vi "Configure Current Limits.vi"(0 "VISA resource name":refnum<visa-resource-name>, 5 "Current Low Limit (0 A)":dbl min=0.0 max=220.8 format="%.3f", 7 "Current High Limit (0 A)":dbl min=0.0 max=220.8 format="%.3f", 9 "Current Type":u16(ring) items=["RMS", "Peak"], 11 "error in (no error)":errorcluster) -> (4 "VISA resource name out":refnum<visa-resource-name>, 15 "error out":errorcluster)   [LabVIEW 2016, in "APT 300XAC Series.lvlib"]
doc: "Configure the current limits in the active step of the power source instrument.\n\n<B>Range</B> : 0.000~55.20 A\n\nAC Mode\nVoltage Range = Low\n310XAC=0.000-9.20\n320XAC=0.000-18.40\n340XAC=0.00-36.80\n360XAC=0.00-55.20\n\nVoltage Range = High\n310XAC=0.000-4.60\n320XAC=0.000-9.20\n340XAC=0.00-18.40\n360XAC=0.00-27.60\n\n\nDC Mode\nVoltage Range = Low\n310XAC=0.000-4.80\n320XAC=0.000-9.60\n340XAC=0.00-19.20\n360XAC=0.00-28.80\n\nVoltage Range = High\n310XAC=0.000-2.40\n320XAC=0.000-4.80\n340XAC=0.00-9.60\n360XAC=0.00-14.40\n\nThe current Limit setting configures a current threshold level. A test failure will occur when the high limit is reached or the low limit is not reached.\n\nNote : This VI can be used only for Program Mode.\nRun \"Configure Program Mode.vi\" to make sure the instrument is in <B>Program Mode</B> before using this VI"
uses:
  APT 300XAC Series.lvlib
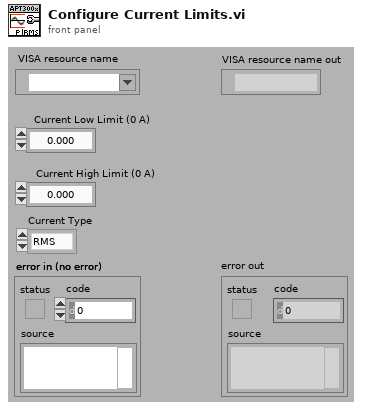
[diagram p1: front panel]
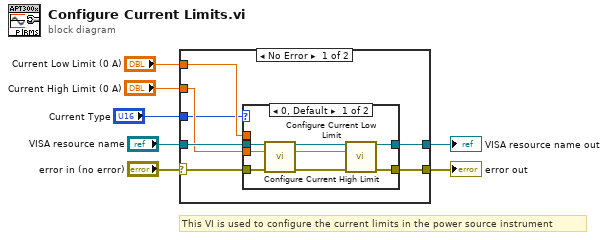
[diagram p0: block diagram]
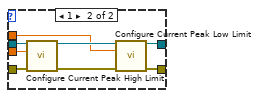
[diagram p2: hidden frame]
diagram:
  # "This VI is used to configure the current limits in the power source instrument"
  n1 = case shown="No Error" "error in (no error)" {
    selector: "error in (no error)" -> [w13 w32]
    tunnel: [w10 w32] -> w7
    tunnel: [w9 w31] -> w6
    tunnel: "VISA resource name" -> [w14 w31]
    tunnel: "Current High Limit (0 A)" -> [w12 _]
    tunnel: "Current Low Limit (0 A)" -> [w11 _]
    tunnel: "Current Type" -> [w8 _]
    frame No Error {
      n2 = case shown="0, Default" w8 {
        tunnel: w14 -> [w20 w29]
        tunnel: w13 -> [w19 w28]
        tunnel: w12 -> [w18 w23]
        tunnel: w11 -> [w17 w24]
        tunnel: [w16 w26] -> w10
        tunnel: [w15 w27] -> w9
        frame 0, Default {
          n3 = call "Configure Current High Limit.vi"("VISA resource name"=w20, "Current High Limit (0 A)"=w18, "error in (no error)"=w19) -> ("VISA resource name out"=w21:refnum<visa-resource-name>, "error out"=w22:errorcluster)  [unwired: 11 in]
          n4 = call "Configure Current Low Limit.vi"("VISA resource name"=w21, "Current Low Limit (0 A)"=w17, "error in (no error)"=w22) -> ("VISA resource name out"=w15:refnum<visa-resource-name>, "error out"=w16:errorcluster)  [unwired: 11 in]
        }
        frame 1 {
          n5 = call "Configure Current Peak High Limit.vi"("VISA resource name"=w29, "Current Peak High Limit (0 A)"=w23, "error in (no error)"=w28) -> ("VISA resource name out"=w30:refnum<visa-resource-name>, "error out"=w25:errorcluster)  [unwired: 11 in]
          n6 = call "Configure Current Peak Low Limit.vi"("VISA resource name"=w30, "Current Peak Low Limit (0 A)"=w24, "Error In"=w25) -> ("VISA resource name out"=w27:refnum<visa-resource-name>, "error out"=w26:errorcluster)  [unwired: 11 in]
        }
      }
    }
    frame Error {
    }
  }
  "error out" <- w7
  "VISA resource name out" <- w6
